vi "PV error_handling.vi"(7 "Data Typ in":string, 8 "error in":errorcluster, 9 "response (data) in":string, 10 "Parameter\nread only<->describe":bool, 11 "data in":string) -> (0 "error out":errorcluster, 2 "Data out":string, 3 "PV Protocol Data out":string)   [LabVIEW 2015, in "Pfeiffer Vacuum.lvlib"]
uses:
  Pfeiffer Vacuum.lvlib
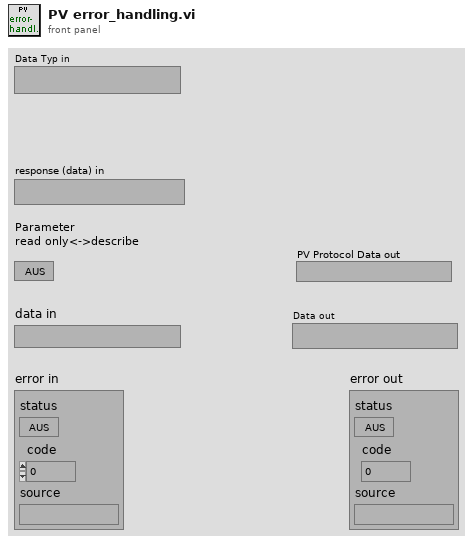
[diagram p1: front panel]
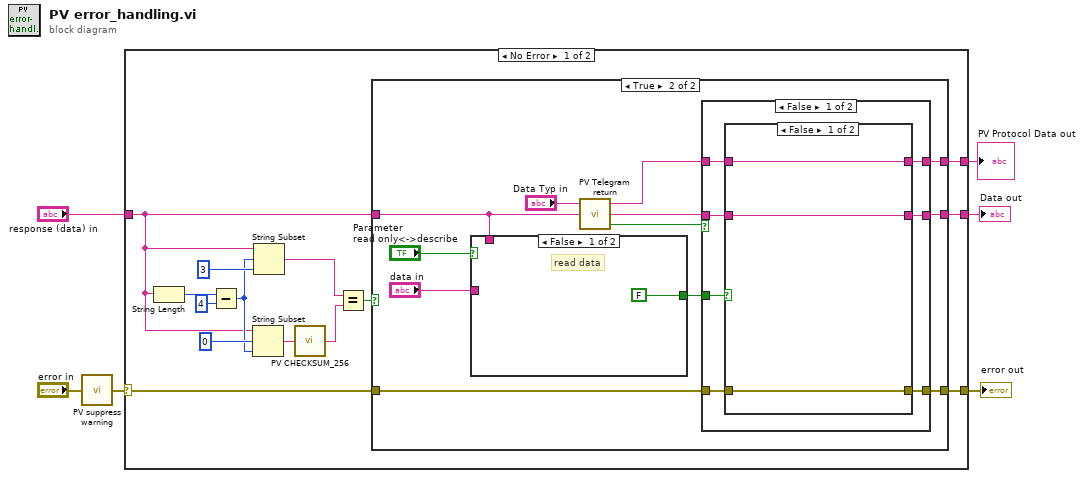
[diagram p0: block diagram]
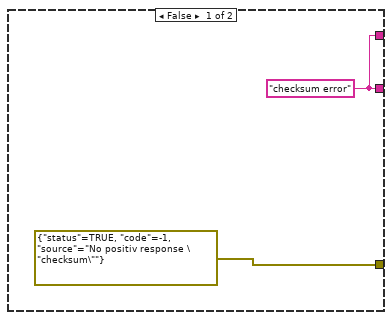
[diagram p2: hidden frame]
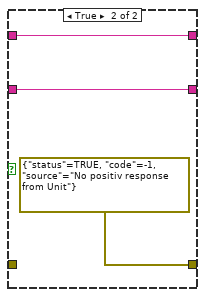
[diagram p3: hidden frame]
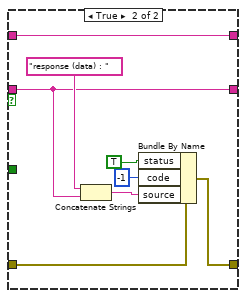
[diagram p4: hidden frame]
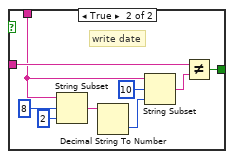
[diagram p5: hidden frame]
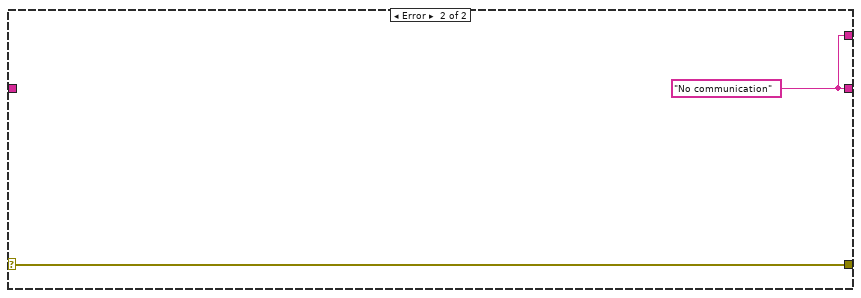
[diagram p6: hidden frame]
diagram:
  n1 = call "PV suppress warning.vi"("error in"="error in") -> ("error out"=w2:errorcluster)
  n2 = case shown="No Error" w2 {
    selector: w2 -> [w8 w67]
    tunnel: [w20 w67] -> w6
    tunnel: "response (data) in" -> [w11 _]
    tunnel: [w9 w66] -> w4
    tunnel: [w7 w66] -> w1
    frame No Error {
      n3 = String Length(string=w11) -> (length=w17:i32)
      n4 = Subtract(x=w17, y=4) -> (x-y=w14:i32)
      n5 = String Subset(string=w11, offset (0)=0 ("Offset (0)"), length (rest)=w14) -> (substring=w13:string)
      n6 = String Subset(string=w11, offset (0)=w14, length (rest)=3 ("Länge (Rest)")) -> (substring=w19:string)
      n7 = call "PV CHECKSUM_256.VI"("input string"=w13) -> ("checksum"=w12:string)
      n8 = Equal?(x=w19, y=w12) -> (x = y?=w10:bool)
      n9 = case shown="True" w10 {
        tunnel: [errorcluster {"status"=TRUE, "code"=-1, "source"="No positiv response \"checksum\""} ("Fehlerausgang") w30] -> w20
        tunnel: w11 -> [_ w25]
        tunnel: w8 -> [_ w26]
        tunnel: [w21 w27] -> w9
        tunnel: [w21 w23] -> w7
        frame False {
          w21 = "checksum error" ("source")
        }
        frame True {
          n10 = case shown="False" "Parameter\nread only<->describe" {
            tunnel: "data in" -> [_ w63]
            tunnel: [FALSE w62] -> w32
            tunnel: w25 -> [_ w59]
            frame False {
              # "read data"
            }
            frame True {
              # "write date"
              n11 = String Subset(string=w59, offset (0)=8 ("Offset (0)"), length (rest)=2 ("Länge (Rest)")) -> (substring=w58:string)
              n12 = Decimal String To Number(string=w58) -> (number=w57:i32)  [unwired: 2 in, 1 out]
              n13 = String Subset(string=w59, offset (0)=10 ("Offset (0)"), length (rest)=w57) -> (substring=w64:string)
              n14 = Not Equal?(x=w63, y=w64) -> (x != y?=w62:bool)
            }
          }
          n15 = call "PV Telegram return.vi"("String received"=w25, "Data Typ String"="Data Typ in") -> ("error"=w29:bool, "Substring"=w31:string, "PV Protocol Data out"=w24:string)  [unwired: 1 in]
          n16 = case shown="False" w29 {
            tunnel: [w41 w55] -> w30
            tunnel: w31 -> [w39 w49]
            tunnel: w32 -> [w40 _]
            tunnel: [w38 w49] -> w27
            tunnel: w26 -> [w37 w50]
            tunnel: w24 -> [w36 w48]
            tunnel: [w35 w48] -> w23
            frame False {
              n17 = case shown="False" w40 {
                tunnel: [w43 errorcluster {"status"=TRUE, "code"=-1, "source"="No positiv response from Unit"} ("Fehlerausgang")] -> w41
                tunnel: w39 -> [w44 w46]
                tunnel: [w44 w46] -> w38
                tunnel: w37 -> [w43 _]
                tunnel: w36 -> [w42 w45]
                tunnel: [w42 w45] -> w35
                frame False {
                }
                frame True {
                }
              }
            }
            frame True {
              n18 = Concatenate Strings("response (data) : " ("Elemente bündeln"), w49) -> (w51:string)
              n19 = Bundle By Name(cluster=w50, "status"=TRUE ("Elemente bündeln"), "code"=-1 ("Elemente bündeln"), "source"=w51) -> (w55:errorcluster)
            }
          }
        }
      }
    }
    frame Error {
      w66 = "No communication" ("y")
    }
  }
  "error out" <- w6
  "Data out" <- w4
  "PV Protocol Data out" <- w1
